vi "Read Update HS Bcklg.vi"(8 "error in (no error)":errorcluster, 11 "FP Controls in":refnum<class "FP Controls.lvclass">) -> (0 "error out":errorcluster, 2 "Update HS Bcklg":refnum<user-event>, 3 "FP Controls out":refnum<class "FP Controls.lvclass">)   [LabVIEW 2012, in "Configuration Grandmaster.lvlib" / "FP Controls.lvclass"]
uses:
  FP Controls.lvclass
  FP Controls.lvclass/FP Controls.ctl
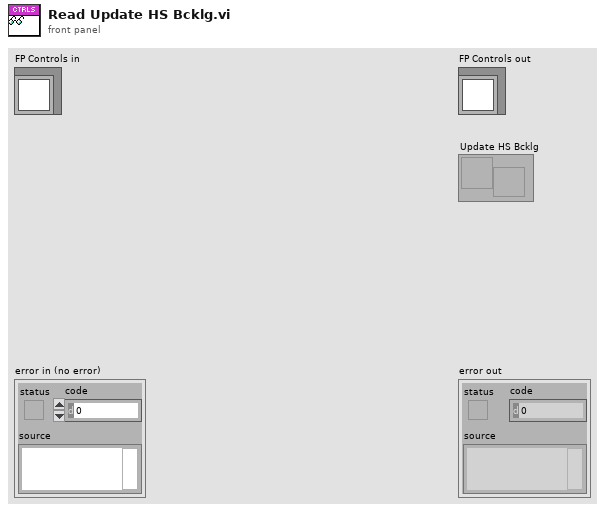
[diagram p1: front panel]
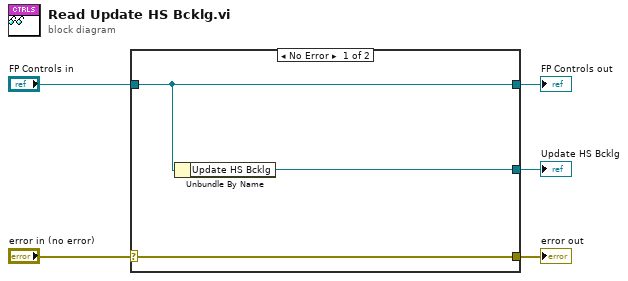
[diagram p0: block diagram]
diagram:
  n1 = case shown="No Error" "error in (no error)" {
    selector: "error in (no error)" -> [w8 w9]
    tunnel: [w8 w9] -> w4
    tunnel: [w7 w10] -> w2
    tunnel: "FP Controls in" -> [w7 w10]
    tunnel: [w6 _] -> w1
    frame No Error {
      n2 = Unbundle By Name(w7) -> ("Update HS Bcklg"=w6:refnum<user-event>)
    }
    frame Error {
    }
  }
  "error out" <- w4
  "FP Controls out" <- w2
  "Update HS Bcklg" <- w1
